vi "Read Disabled count.vi"(11 "Test Suite Result In":refnum<class "Test Suite Result.lvclass">) -> (1 "Disabled count string":string, 2 "Disabled count":i32, 3 "Test Suite Result Out":refnum<class "Test Suite Result.lvclass">)   [LabVIEW 2020, in "Test Suite Result.lvclass"]
uses:
  Test Suite Result.lvclass
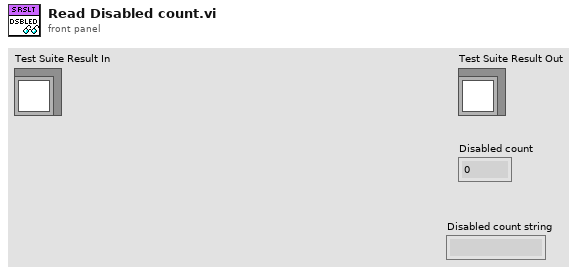
[diagram p1: front panel]
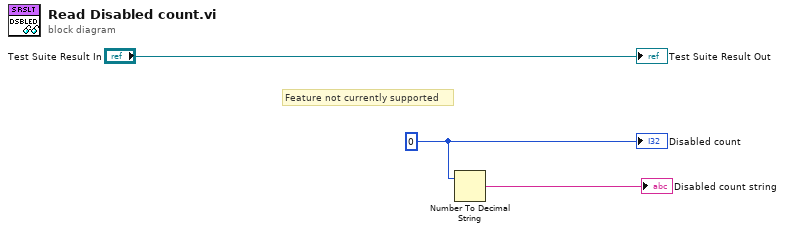
[diagram p0: block diagram]
diagram:
  w1 = 0 ("Disabled count")
  # "Feature not currently supported"
  n1 = Number To Decimal String(number=w1) -> (decimal integer string=→"Disabled count string":string)  [unwired: 1 in]
  "Test Suite Result Out" <- "Test Suite Result In"
  "Disabled count" <- w1
